vi "SetSpectrometerIntegrationTime.vi"(8 "error in (no error)":errorcluster, 10 "Integration Time (ms)":i32=80, 11 "StellarNetSpecAcquisition in":refnum<class "StellarNetSpecAcquisition.lvclass">) -> (0 "error out":errorcluster, 3 "StellarNetSpecAcquisition out":refnum<class "StellarNetSpecAcquisition.lvclass">)   [LabVIEW 2020, in "StellarNetSpecAcquisition.lvclass"]
uses:
  StellarNetSpecAcquisition.lvclass
  StellarNetSpectrometer.lvclass
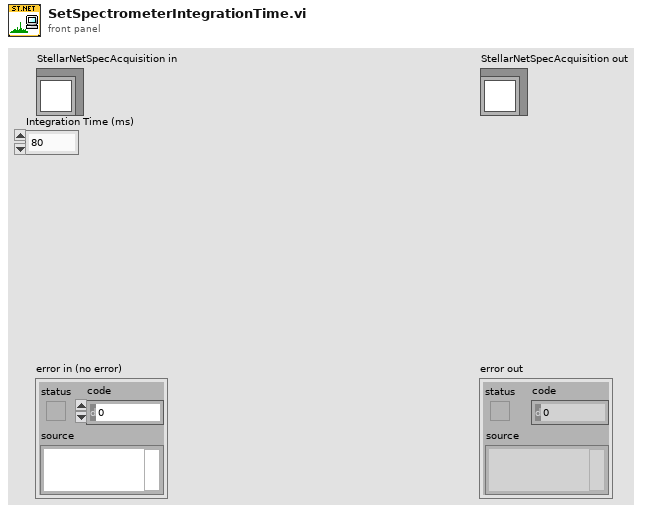
[diagram p1: front panel]
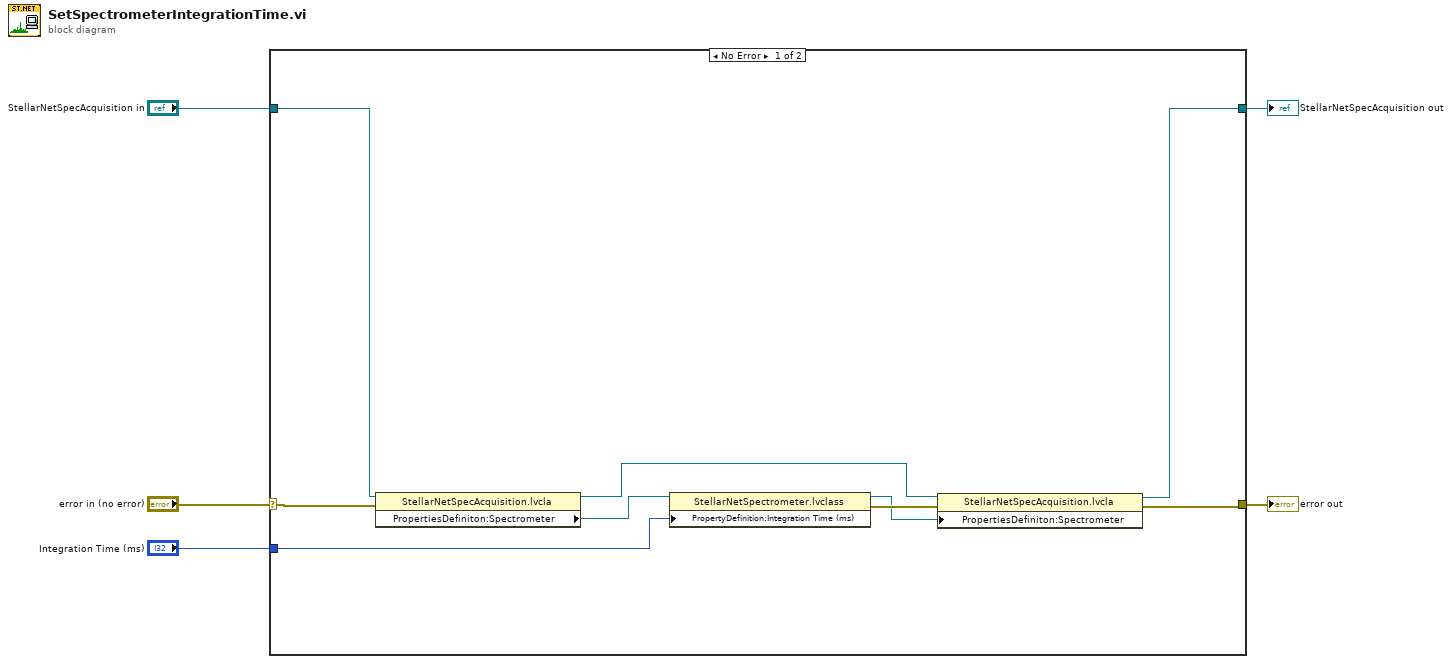
[diagram p0: block diagram]
diagram:
  n1 = case shown="No Error" "error in (no error)" {
    selector: "error in (no error)" -> [w10 w16]
    tunnel: [w8 w16] -> w4
    tunnel: [w6 w15] -> w2
    tunnel: "StellarNetSpecAcquisition in" -> [w7 w15]
    tunnel: "Integration Time (ms)" -> [w9 _]
    frame No Error {
      n2 = property class="StellarNetSpecAcquisition.lvcla"(reference=w7, error in=w10) -> (reference out=w14:refnum<class "StellarNetSpecAcquisition.lvclass">, "PropertiesDefiniton:Spectrometer"=w11:refnum<class "StellarNetSpectrometer.lvclass">)  [unwired: 1 out]
      n3 = property class="StellarNetSpectrometer.lvclass"(reference=w11, "PropertyDefinition:Integration Time (ms)"=w9) -> (reference out=w12:refnum<class "StellarNetSpectrometer.lvclass">, error out=w13:errorcluster)  [unwired: 1 in]
      n4 = property class="StellarNetSpecAcquisition.lvcla"(reference=w14, error in=w13, "PropertiesDefiniton:Spectrometer"=w12) -> (reference out=w6:refnum<class "StellarNetSpecAcquisition.lvclass">, error out=w8:errorcluster)
    }
    frame Error {
    }
  }
  "error out" <- w4
  "StellarNetSpecAcquisition out" <- w2
